vi "flattenTimeToXML.vi"   [LabVIEW 2012, in "UnitsAndXML.lvlib"]
doc: "Generates an XML string for <B>time</B> in the unit specified in <B>timeUnitInXML</B>. Connect <B>time</B> and <B>timeAgain</B> to the same source. The VI uses <B>timeAgain</B> to obtain the data name."
uses:
  <userlib>/Common/UnitsAndXML/UnitsAndXML.lvlib
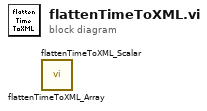
[diagram p0: block diagram]
diagram:
  n1 = call <userlib>:"flattenTimeToXML_Array.vi"() -> ()  [unwired: 10 in, 2 out]
  n2 = call <userlib>:"flattenTimeToXML_Scalar.vi"() -> ()  [unwired: 10 in, 2 out]
